vi "Bind Listbox Item Names.vi"(8 "error in (no error)":errorcluster, 9 "Datum Name (\"\"=Use Control Label)":string, 10 "LstBox Refnum":refnum<vi>, 11 "IViewable in":refnum<class "IViewable.lvclass">) -> (0 "error out":errorcluster, 3 "IViewable out":refnum<class "IViewable.lvclass">)   [LabVIEW 2017, in "IViewable.lvlib" / "IViewable.lvclass"]
doc: "Bind the Item Names of a single-column listbox to an published 1-D array of strings."
uses:
  IViewable.lvclass
  C:/Program Files (x86)/National Instruments/LabVIEW 2017/vi.lib/ActorFramework/Actor/Actor.lvclass
  <vilib>/ActorFramework/Actor/Actor.lvclass/Actor.ctl
  <vilib>/ActorFramework/Message Enqueuer/Message Enqueuer.lvclass/Message Enqueuer.ctl
  Transport/ListboxItemNamesBinding/ListboxItemNamesBinding.lvclass/ListboxItemNamesBinding.ctl
  SubscriptionPolicy/ValueChangeSubscription/ValueChangeSubscription.lvclass/ValueChangeSubscription.ctl
  IMediator/SubscriptionRequest/SubscriptionRequest.lvclass/SubscriptionRequest.ctl
  IObserver/IObserver Messages/Subscribe Msg/Subscribe Msg.lvclass/Subscribe Msg.ctl
  <vilib>/ActorFramework/Message Enqueuer/Init from Existing Queue.vi
  <vilib>/ActorFramework/Message Enqueuer/Enqueue.vi
  SubscriptionPolicy/ValueChangeSubscription/ValueChangeSubscription.lvclass
  C:/Git/mva-framework/Source/Framework/IMediator/ISubscriptionPolicy/ISubscriptionPolicy.lvclass
  Transport/ListboxItemNamesBinding/ListboxItemNamesBinding.lvclass
  C:/Git/mva-framework/Source/Framework/IMediator/ITransport/ITransport.lvclass
  IObserver/IObserver Messages/Subscribe Msg/Subscribe Msg.lvclass
  C:/Program Files (x86)/National Instruments/LabVIEW 2017/vi.lib/ActorFramework/Message/Message.lvclass
  <vilib>/ActorFramework/Message Priority Queue/Priority Enqueue.vi
  <vilib>/ActorFramework/Message Enqueuer/Message Enqueuer.lvclass
  IMediator/SubscriptionRequest/SubscriptionRequest.lvclass
  <vilib>/ActorFramework/Actor/Actor.lvclass
  IMediator/ISubscriptionPolicy/ISubscriptionPolicy.lvclass
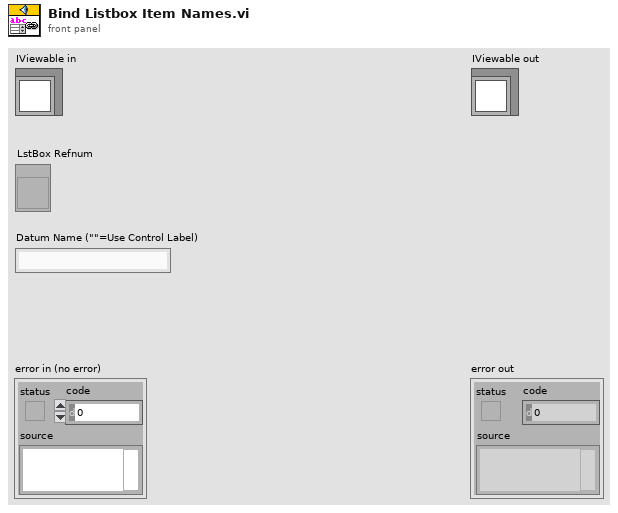
[diagram p1: front panel]
types:
  T1 = typedef "IMediator.lvlib/ISubscriptionPolicy.lvclass/ISubscriptionPolicy Reference.ctl" = refnum<data-value>
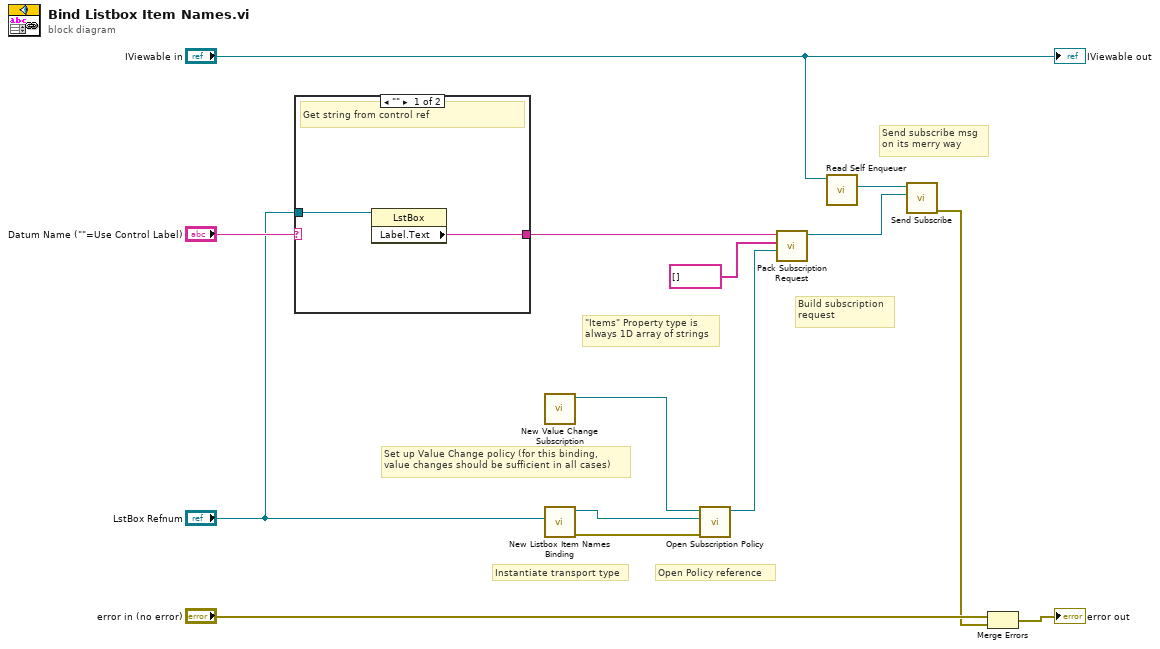
[diagram p0: block diagram]
diagram:
  # "\"Items\" Property type is\nalways 1D array of strings"
  # "Open Policy reference"
  # "Set up Value Change policy (for this binding,\nvalue changes should be sufficient in all cases)"
  # "Send subscribe msg\non its merry way"
  # "Build subscription\nrequest"
  # "Instantiate transport type"
  n1 = case shown="\"\"" "Datum Name (\"\"=Use Control Label)" {
    selector: "Datum Name (\"\"=Use Control Label)" -> [_ w17]
    tunnel: [w15 w17] -> w8
    tunnel: "LstBox Refnum" -> [w16 _]
    frame "" {
      # "Get string from control ref"
      n2 = property class="LstBox"(reference=w16) -> ("Label.Text"=w15:string)  [unwired: 1 in, 2 out]
    }
    frame Default {
      # "Use string wired to input terminal"
    }
  }
  n3 = call "New Value Change Subscription.vi"() -> ("ValueChangeSubscription Out"=w4:refnum<class "ValueChangeSubscription.lvclass">)  [unwired: 11 in]
  n4 = call "New Listbox Item Names Binding.vi"("LstBox Refnum"="LstBox Refnum") -> ("error out"=w3:errorcluster, "MCListboxItemNamesBinding"=w6:refnum<class "ListboxItemNamesBinding.lvclass">)  [unwired: 9 in]
  n5 = call "Open Subscription Policy.vi"("error in (no error)"=w3, "Transport"=w6, "SubscriptionPolicy"=w4) -> ("Subscription Policy"=w1:T1)  [unwired: 7 in, 1 out]
  n6 = call "Pack Subscription Request.vi"("Subscription Policy"=w1, "Type"=string[] [], "Datum Name"=w8) -> ("SubscriptionRequest"=w5:refnum<class "SubscriptionRequest.lvclass">)  [unwired: 8 in]
  n7 = call <vilib>:"Read Self Enqueuer.vi"("Actor"="IViewable in") -> ("Self Enqueuer"=w12:refnum<class "Message Enqueuer.lvclass">)  [unwired: 10 in]
  n8 = call "Send Subscribe.vi"("SubscriptionRequest"=w5, "Message Enqueuer"=w12) -> ("error out"=w10:errorcluster)  [unwired: 8 in, 1 out]
  n9 = Merge Errors("error in (no error)", w10) -> (→"error out":errorcluster)
  "IViewable out" <- "IViewable in"
